vi "Modules - Communications V2-multiple.vi"() -> ()   [LabVIEW 2019]
uses:
  Controls/UDP - Event.ctl
  Controls/UDP - Status.ctl
  Controls/Communications - State.ctl
  Controls/UDP - Command.ctl
  Controls/eFGV States.ctl
  Controls/Communications - Data Structure.ctl
  Controls/FTDI - Communication.ctl
  Controls/Communication - Write Data.ctl
  Controls/UDP - Communication.ctl
  Controls/Global - Hold.vi
  Controls/Global - IP Address.vi
  Controls/Global - Handle.vi
  Controls/Global - Comport.vi
  Controls/Global - Device.vi
  Controls/Global - Data UDP.vi
  Controls/Global - Device Type.vi
  Controls/Global - Unit.vi
  Controls/Global - ADC.vi
  Controls/Global - PID.vi
  Controls/Global - System.vi
  Controls/Global - Test.vi
  Controls/Global - Channel.vi
  Controls/Global - Rendezvous.vi
  Controls/FGV States.ctl
panel:
  out "element":string
  out "UI Loop":errorcluster
  out "UDP CMD.CMD":T1
  out "Feed Error":errorcluster
  out "i Feed Loop":i32
  out "Feed Loop":T2
  out "i CMD Loop":i32
  out "CMD Loop":T2
  out "i UI Loop":i32
  out "UI Loop":T2
  out "CMD Addr":T3
  out "IP":string
  out "IP Registered":string[](array[string])
  out "Array":cluster{"error out":errorcluster, "IP":string}[](array[cluster])
  out "error out":errorcluster
  in  "timeout ms":i32=1000
  out "data out":string
  out "Array 2":T6(array[cluster]) {"Data"."Event" items=["Stop", "Running", "PID", "Up Limit", "Down Limit", "Load Limit"]; "Data"."Status" items=["Stop", "Ramp Up", "Ramp Down", "Jog Up", "Jog Down", "PID Mode", "PID Ramp"]}
  out "UDP Conn ref":refnum<k16>
  out "Stop":bool=TRUE
  out "IP":string[](array[string])
  out "Device":string[](array[string])
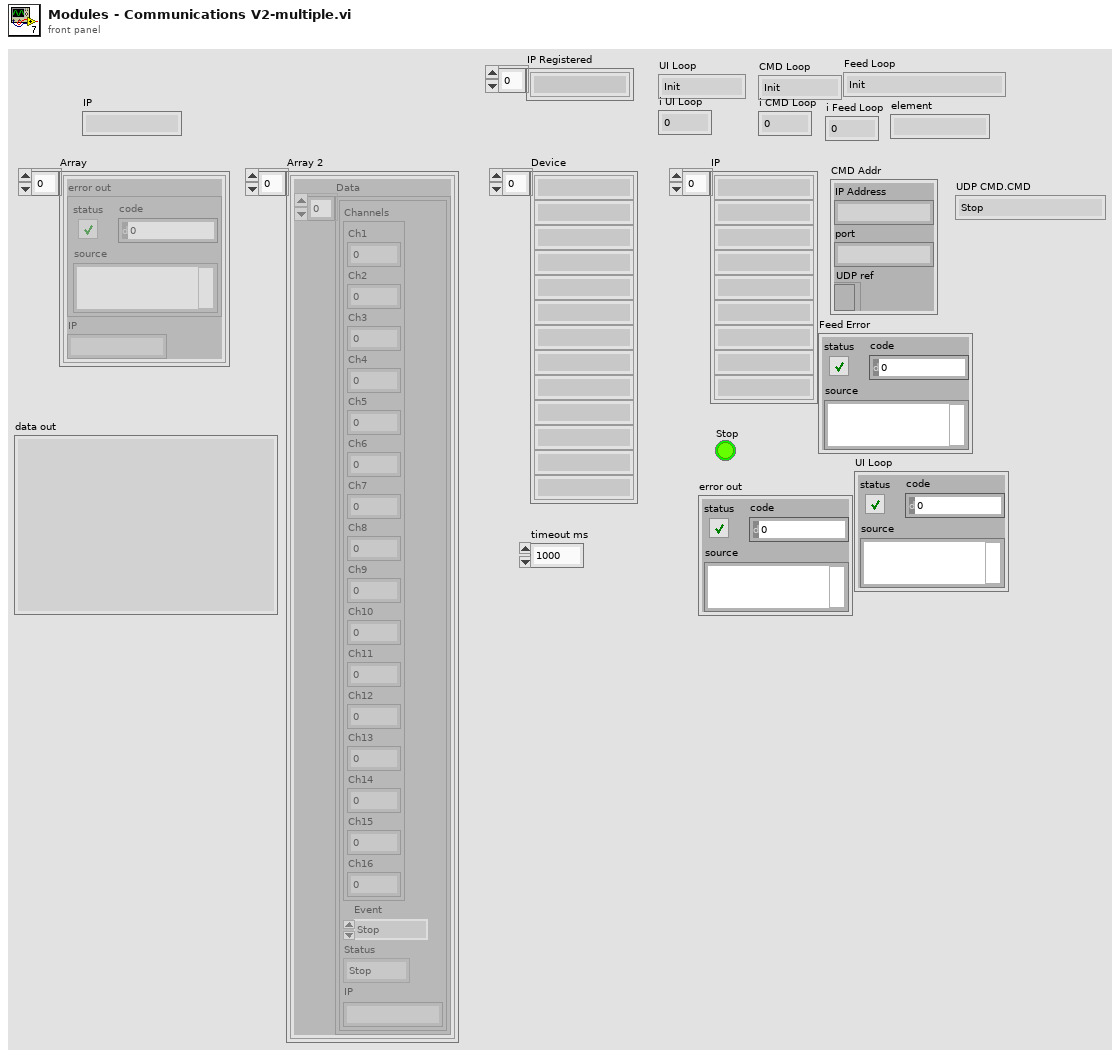
[diagram p1: front panel]
types:
  T1 = typedef "UDP - Command.ctl" = enum16{"Stop", "Jog Up", "Jog Down", "Ramp Up", "Ramp Down", "PID Target", "PID Ramp", "Disp Run", "Read Ch Data", "Zero Channel", "Zero Disp", "Read Sensor", "Write Sensor", "Read ADC", "Write ADC", "Read PID", "Write PID", "Read Test", "Write Test", "Read System", "Write System", "Read Datalog", "Read Datalog Sensor"}
  T2 = typedef "Communications - State.ctl" = enum16{"Init", "Idle", "Command", "Get IP Address", "Release Rendezvous", "Feedback", "Close"}
  T3 = cluster{"IP Address":string, "port":string, "UDP ref":refnum<k16>}
  T4 = typedef "UDP - Event.ctl" = u16
  T5 = typedef "UDP - Status.ctl" = u16
  T6 = cluster{"Data":cluster{"Channels":cluster{"Ch1":sgl, "Ch2":sgl, "Ch3":sgl, "Ch4":sgl, "Ch5":sgl, "Ch6":sgl, "Ch7":sgl, "Ch8":sgl, "Ch9":sgl, "Ch10":sgl, "Ch11":sgl, "Ch12":sgl, "Ch13":sgl, "Ch14":sgl, "Ch15":sgl, "Ch16":sgl}, "Event":T4, "Status":T5, "IP":string}[]}[]
  T7 = cluster{"error out":errorcluster, "name":string}[]
  T8 = enum32{"Invalid", "Standard", "Closed", "Hidden", "Minimized", "Maximized"}
  T9 = typedef "eFGV States.ctl" = enum16{"Init", "Read", "Write", "Exit"}
  T10 = typedef "Communications - Data Structure.ctl" = cluster{"UDP CMD":T11, "Unit?":bool, "Read Unit":bool[], "Trig?":bool, "UDP Info":cluster{"IP Address":string, "port":string, "UDP ref":refnum<k16>}[], "DataLogger":bool[], "VISA Ref":refnum<event-registration>, "Float":sgl, "Data":T12, "UDP Event Ref":refnum<event-registration>, "UDP ref":refnum<k16>, "Read Sensor":u8}
  T11 = typedef "FTDI - Communication.ctl" = cluster{"IP":string, "CMD":T1, "Port":string, "Datalog?":bool, "Float":dbl}
  T12 = typedef "Communication - Write Data.ctl" = cluster{"Test":cluster{"Target Load":sgl, "Target Disp":sgl, "Rate":sgl, "Speed":sgl}, "Sensor":cluster{"Name":string[], "Unit":string[], "Decimal Point":u8[], "Ch Log":u8[], "H Alarm":u8[], "L Alarm":u8[], "H Limit":sgl[], "L Limit":sgl[], "Filter":u8[], "Gain":u8[], "Calib Type":u32[]}, "PID":cluster{"SP":sgl, "PV":sgl, "kP":sgl, "kI":sgl, "kD":sgl, "FF":sgl, "Err Band":sgl, "Max":i32, "Min":i32, "Ts":u32, "Out":i32, "Mode":u8}, "ADC":cluster{"Active Ch":u8[], "Filter Type":u8, "Post Filter":u8[], "Gain":u8[], "FS":u16, "IntOC":u8, "IntFC":u8, "SysOC":u8, "Cofficient":dbl[], "K":dbl[], "Max":i32}, "System":cluster{"Out Type":u8, "Inverse":u8, "Monitor":u8, "Reserve":u8, "ACC Time":u32, "Pulse Rev":u32, "Stroke":u32, "Auto Off":u32, "Gear Ratio":sgl, "Pitch":sgl, "Max Speed":u32, "Jog Speed":u32, "Disp Coff":sgl, "Max Load":u32}, "Index":enum16{"Ch1", "Ch2", "Ch3", "Ch4", "Ch5", "Ch6", "Ch7", "Ch8", "Ch9", "Ch10", "Ch11", "Ch12", "Ch13", "Ch14", "Ch15", "Ch16"}, "Datalog":enum16{"Ch1-Ch16", "Ch17-Ch32", "Ch32-Ch48", "Ch49-Ch64", "Empty"}}
  T13 = enum16{"Ch1-Ch16", "Ch17-Ch32", "Ch32-Ch48", "Ch49-Ch64", "Empty"}
  T14 = cluster{"IP Address":string, "port":string, "UDP ref":refnum<k16>}[]
  T15 = typedef "FGV States.ctl" = enum16{"Read", "Write"}
  T16 = cluster{"Target Load":sgl, "Target Disp":sgl, "Rate":sgl, "Ch4":sgl}
  T17 = cluster{"Name":string[], "Unit":string[], "Decimal Point":u8[], "Ch Log":u8[], "H Alarm":u8[], "L Alarm":u8[], "H Limit":sgl[], "L Limit":sgl[], "Filter":u8[], "Gain":u8[], "Calib Type":u32[]}
  T18 = cluster{"SP":sgl, "PV":sgl, "kP":sgl, "kI":sgl, "kD":sgl, "FF":sgl, "Err Band":sgl, "Max":i32, "Min":i32, "Ts":u32, "Out":i32, "Mode":u8}
  T19 = cluster{"Active Ch":u8[], "Filter Type":u8, "Post Filter":u8[], "Gain":u8[], "FS":u16, "IntOC":u8, "IntFC":u8, "SysOC":u8, "Cofficient":dbl[], "K":dbl[], "Max":i32}
  T20 = cluster{"Out Type":u8, "Inverse":u8, "Monitor":u8, "Reserve":u8, "ACC Time":u32, "Pulse Rev":u32, "Stroke":u32, "Auto Off":u32, "Gear Ratio":sgl, "Pitch":sgl, "Max Speed":u32, "Jog Speed":u32, "Disp Coff":sgl, "Max Load":u32}
  T21 = cluster{"error IO":errorcluster, "name":string}[]
  T22 = cluster{"Name":string[], "Unit":string[], "Decimal Point":u8[], "Ch Log":u8[], "H Alarm":u8[], "L Alarm":u8[], "H Limit":sgl[], "L Limit":sgl[], "Filter":u8[], "Gain":u8[], "Calib Type":u32[]}[]
  T23 = cluster{"Active Ch":u8[], "Filter Type":u8, "Post Filter":u8[], "Gain":u8[], "FS":u16, "IntOC":u8, "IntFC":u8, "SysOC":u8, "Cofficient":dbl[], "K":dbl[], "Max":i32}[]
  T24 = cluster{"SP":sgl, "PV":sgl, "kP":sgl, "kI":sgl, "kD":sgl, "FF":sgl, "Err Band":sgl, "Max":i32, "Min":i32, "Ts":u32, "Out":i32, "Mode":u8}[]
  T25 = cluster{"Out Type":u8, "Inverse":u8, "Monitor":u8, "Reserve":u8, "ACC Time":u32, "Pulse Rev":u32, "Stroke":u32, "Auto Off":u32, "Gear Ratio":sgl, "Pitch":sgl, "Max Speed":u32, "Jog Speed":u32, "Disp Coff":sgl, "Max Load":u32}[]
  T26 = cluster{"Target Load":sgl, "Target Disp":sgl, "Rate":sgl, "Speed":sgl}
  T27 = cluster{"Target Load":sgl, "Target Disp":sgl, "Rate":sgl, "Speed":sgl}[]
  T28 = cluster{"Channels":cluster{"Ch1":sgl, "Ch2":sgl, "Ch3":sgl, "Ch4":sgl, "Ch5":sgl, "Ch6":sgl, "Ch7":sgl, "Ch8":sgl, "Ch9":sgl, "Ch10":sgl, "Ch11":sgl, "Ch12":sgl, "Ch13":sgl, "Ch14":sgl, "Ch15":sgl, "Ch16":sgl}, "Event":T4, "Status":T5, "IP":string}[]
  T29 = cluster{"Data":cluster{"Channels":cluster{"Ch1":sgl, "Ch2":sgl, "Ch3":sgl, "Ch4":sgl, "Ch5":sgl, "Ch6":sgl, "Ch7":sgl, "Ch8":sgl, "Ch9":sgl, "Ch10":sgl, "Ch11":sgl, "Ch12":sgl, "Ch13":sgl, "Ch14":sgl, "Ch15":sgl, "Ch16":sgl}, "Event":T4, "Status":T5, "IP":string}[]}
  T30 = typedef "Rendezvous RefNum" = refnum<k1>
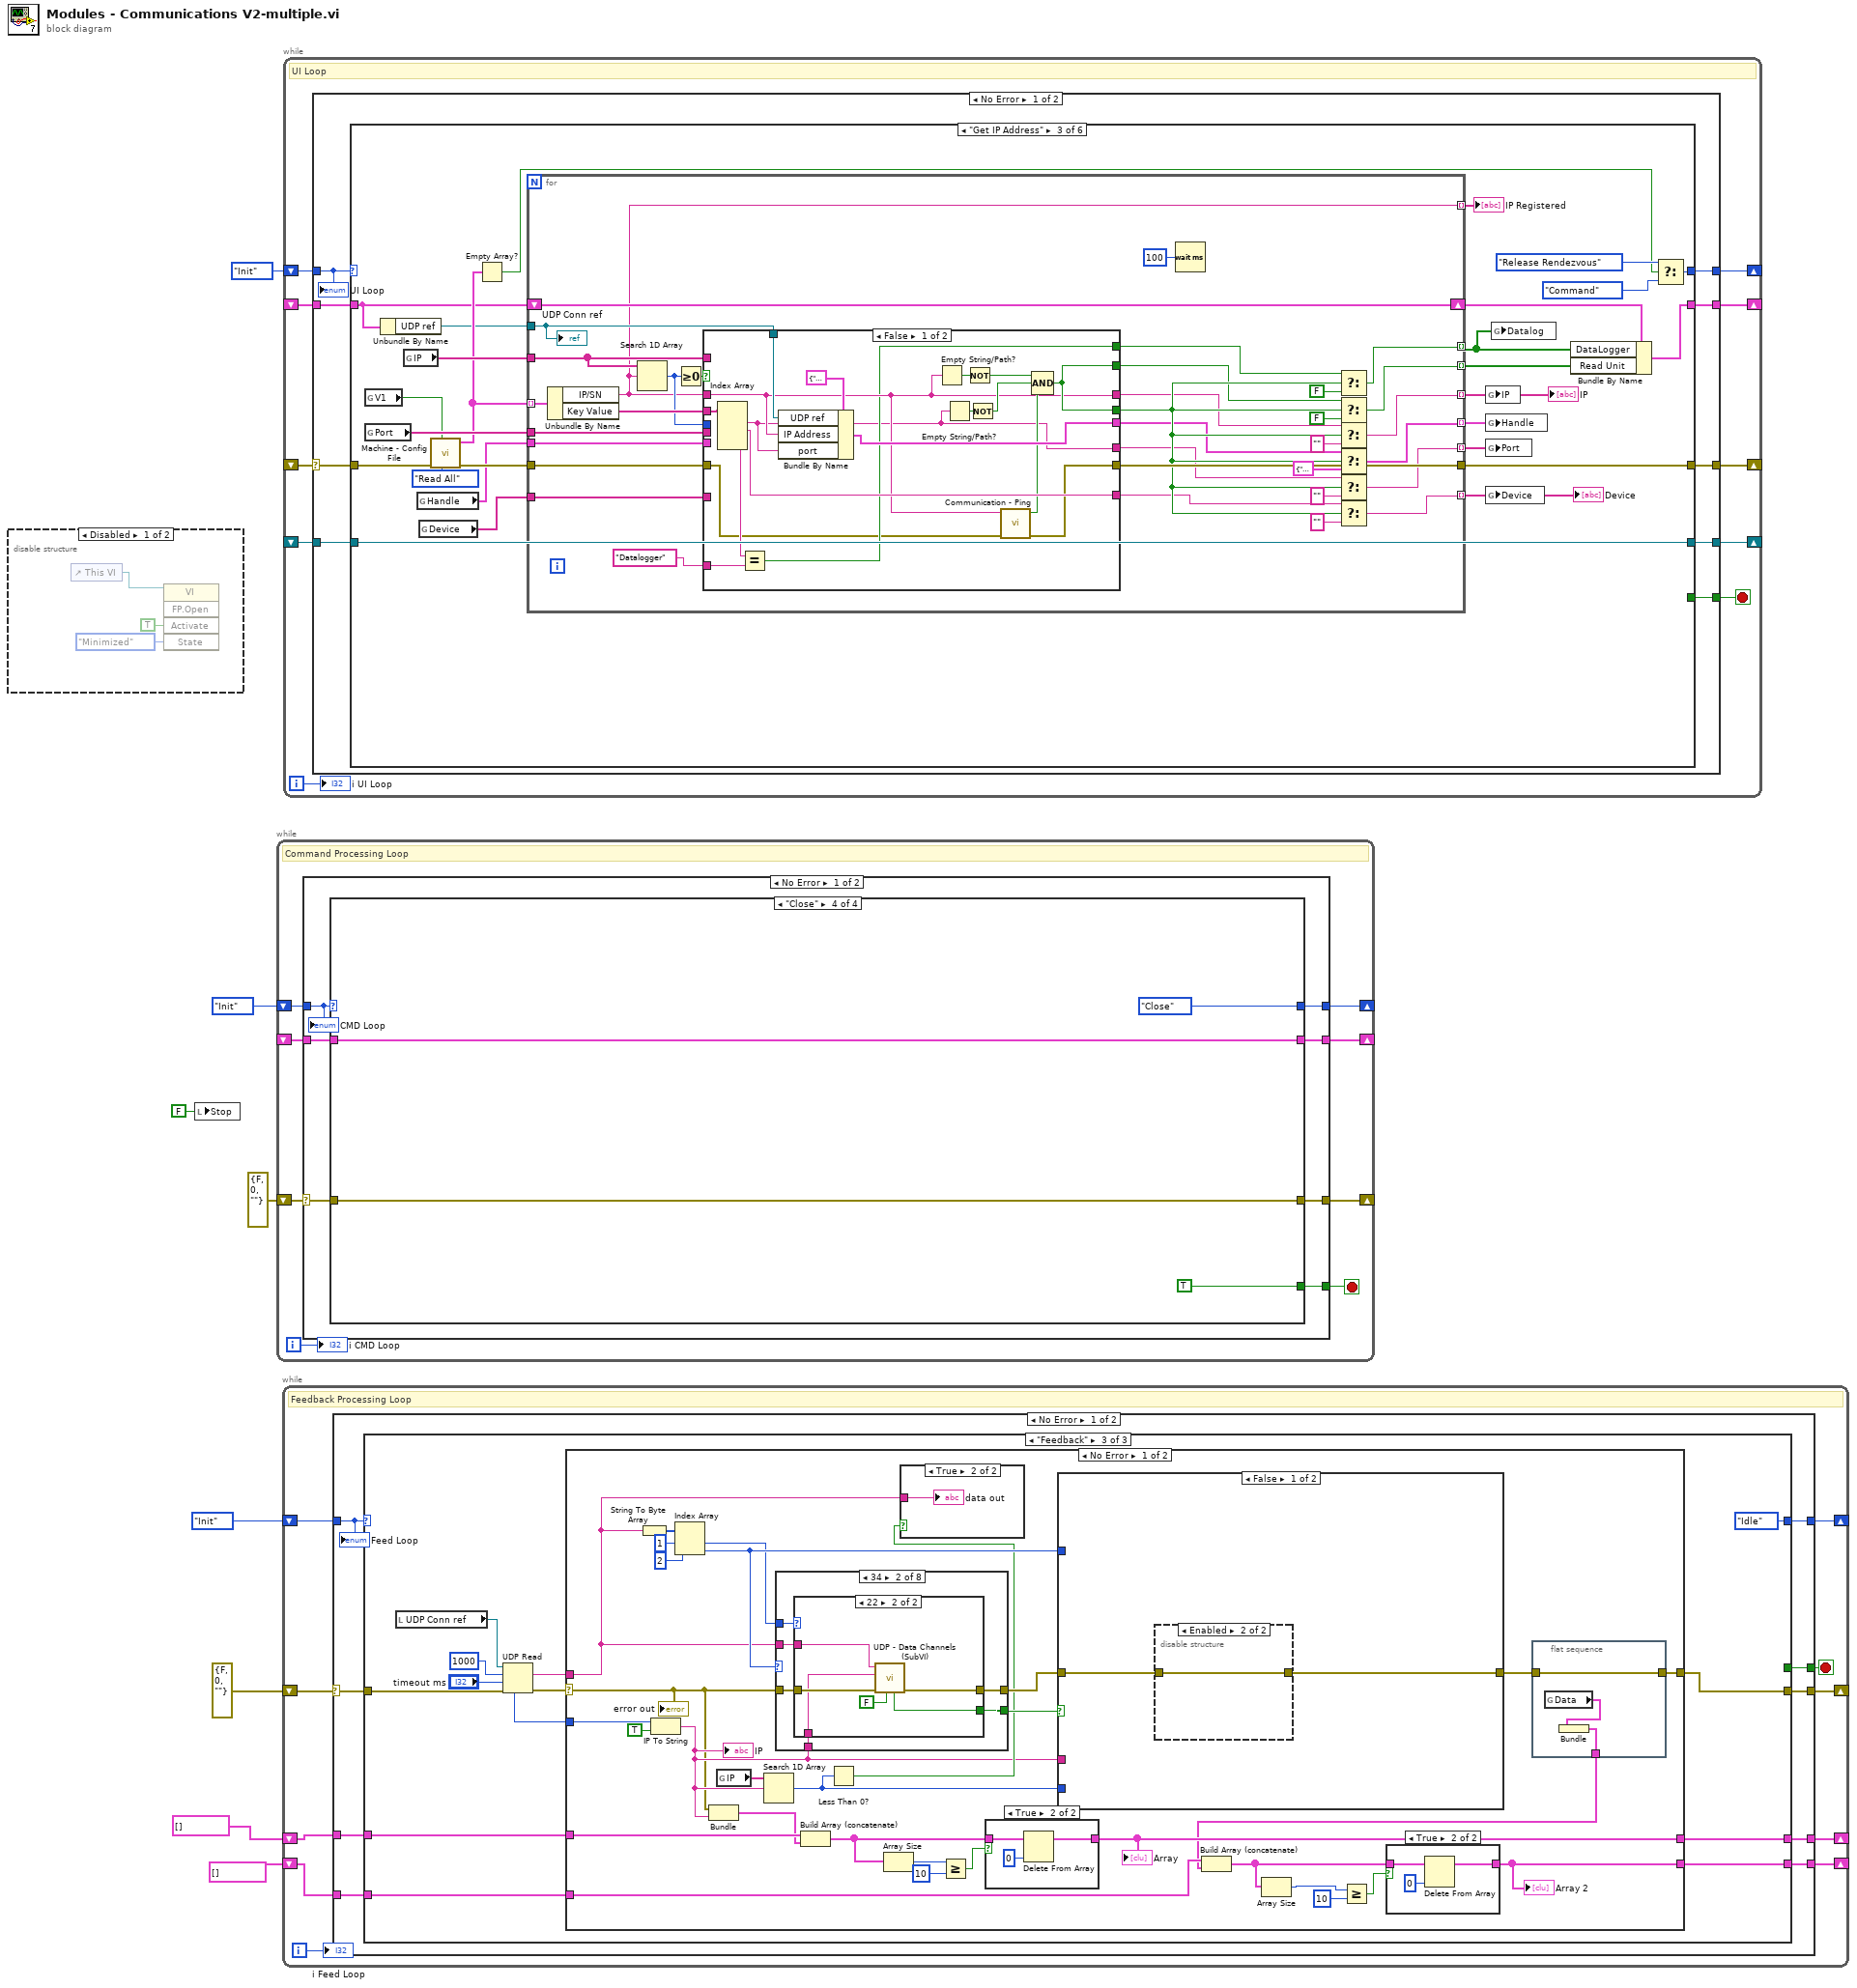
[diagram p0: block diagram]
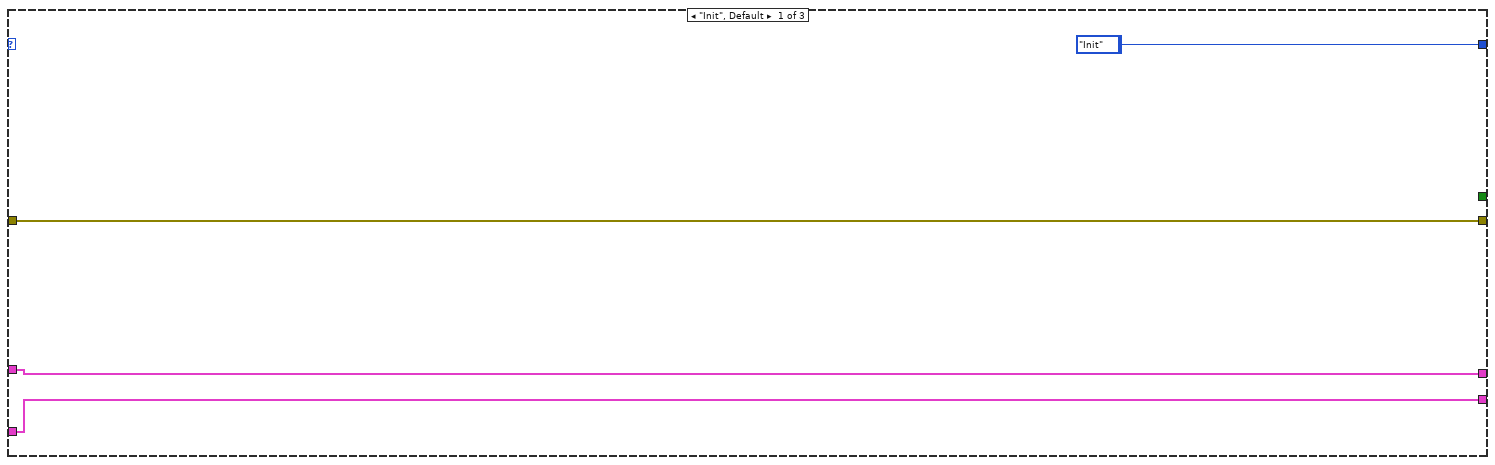
[diagram p3: hidden frame]
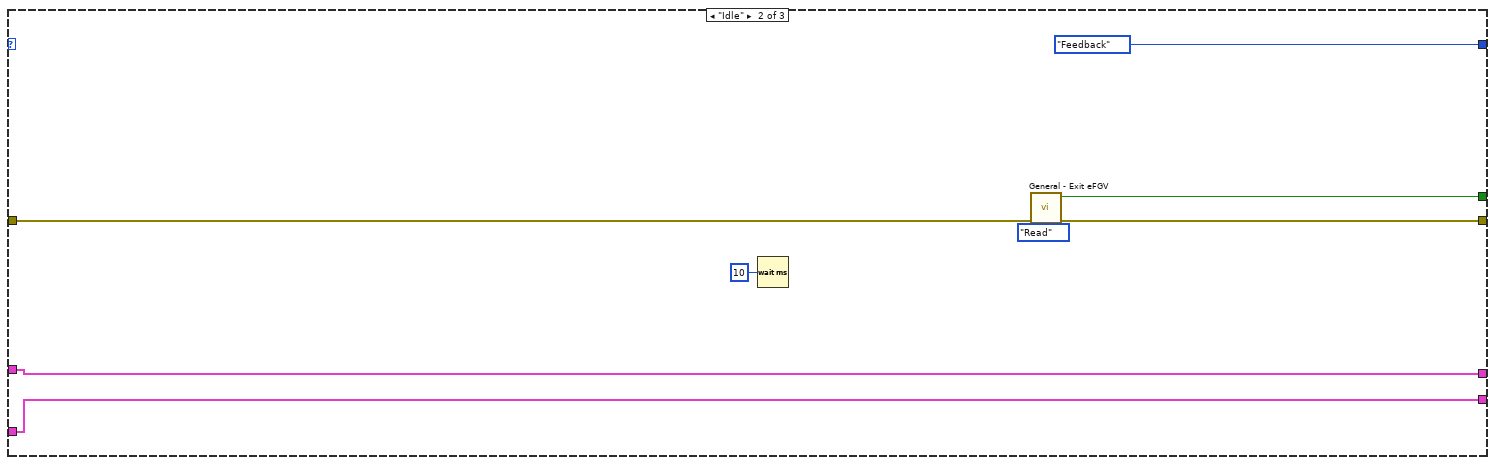
[diagram p4: hidden frame]
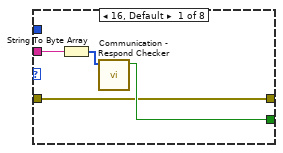
[diagram p8: hidden frame]
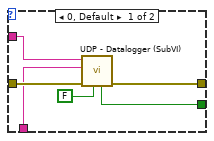
[diagram p9: hidden frame]
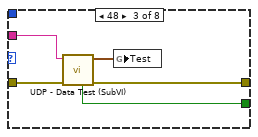
[diagram p10: hidden frame]
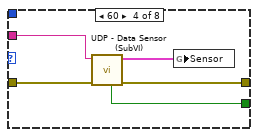
[diagram p11: hidden frame]
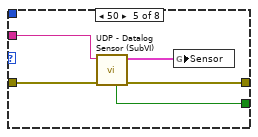
[diagram p12: hidden frame]
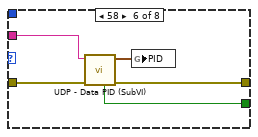
[diagram p13: hidden frame]
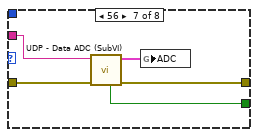
[diagram p14: hidden frame]
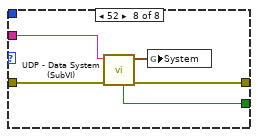
[diagram p15: hidden frame]
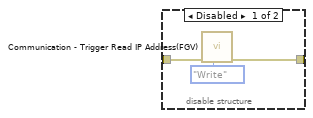
[diagram p16: hidden frame]
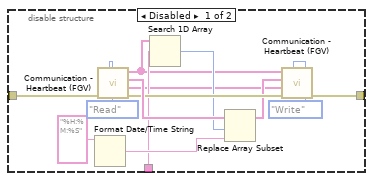
[diagram p19: hidden frame]
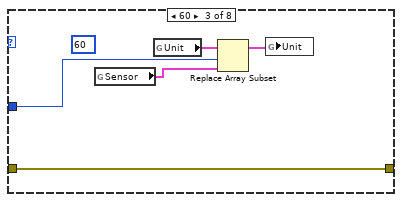
[diagram p20: hidden frame]
diagram:
  (unwired) Communications_-_State."Init"
  (unwired) Communications_-_State."Init"
  n1 = disable-structure shown="Disabled" {
    frame Disabled {
      n2 = control-ref of="This VI"() -> (w11:refnum<vi>)
      n3 = invoke class="VI" method="FP.Open"(reference=w11, "Activate"=TRUE ("Activate?"), "State"=T8."Minimized") -> ()  [unwired: 2 in, 5 out]
    }
    frame Enabled {
    }
  }
  n4 = local write "Stop"(FALSE ("Stop")) -> ()
  n5 = while {
    shift-right: [w18] -> _
    shift-left: errorcluster {"status"=FALSE, "code"=0, "source"=""} ("error IO") -> [w19]
    shift-right: [w16] -> _
    shift-left: Communications_-_State."Init" -> [w17]
    shift-right: [w14] -> _
    shift-left: _ -> [w13]
    i -> [w12]
    stop <- w15 stop-if-true
    # "Command Processing Loop"
    n6 = case shown="No Error" w19 {
      selector: w19 -> [w25 w109]
      tunnel: [w26 w102] -> w18
      tunnel: w17 -> [w24 _]
      tunnel: [w23 Communications_-_State."Idle"] -> w16
      tunnel: [w22 _] -> w15
      tunnel: [w21 w111] -> w14
      tunnel: w13 -> [w20 w111]
      frame No Error {
        n7 = case shown="\"Close\"" w24 {
          tunnel: [w30 w44 w78 w99] -> w26
          tunnel: w25 -> [w28 w43 w88 w99]
          tunnel: [Communications_-_State."Idle" w38 Communications_-_State."Idle" Communications_-_State."Close"] -> w23
          tunnel: [_ _ _ TRUE] -> w22
          tunnel: [w32 w42 w87 w96] -> w21
          tunnel: w20 -> [_ w41 w87 w96]
          frame "Init", Default {
            n8 = call "Communication - UDP Command (eFGV).vi"("Action"=eFGV_States."Read", "error in"=w28) -> ("error out"=w31:errorcluster, "UDP Ref"=w29:refnum<user-event>)  [unwired: 7 in, 1 out]
            n9 = register-events(error in=w31, w29) -> (reference out=w27:refnum<event-registration>, error out=w30:errorcluster)  [unwired: 1 in]
            n10 = Bundle By Name(cluster=T10 {"UDP CMD"={"IP"="", "CMD"=enum."Stop", "Port"="", "Datalog?"=FALSE, "Float"=0.0}, "Unit?"=FALSE, "Read Unit"=[], "Trig?"=FALSE, "UDP Info"=[], "DataLogger"=[], "VISA Ref"=refnum, "Float"=0.0, "Data"={"Test"={"Target Load"=0.0, "Target Disp"=0.0, "Rate"=0.0, "Speed"=0.0}, "Sensor"={"Name"=[], "Unit"=[], "Decimal Point"=[], "Ch Log"=[], "H Alarm"=[], "L Alarm"=[], "H Limit"=[], "L Limit"=[], "Filter"=[], "Gain"=[], "Calib Type"=[]}, "PID"={"SP"=-2.7823365e-08, "PV"=-3.023652e-13, "kP"=8.5432666e-24, "kI"=2.29252e-41, "kD"=1.570387e-38, "FF"=25.0, "Err Band"=0.0, "Max"=15, "Min"=-7, "Ts"=1886611780, "Out"=0, "Mode"=0}, "ADC"={"Active Ch"=[255, 255, 255, 0, 0, 0, 0, 0], "Filter Type"=2, "Post Filter"=[1, 1, 1, 1, 0, 200, 66, 184], "Gain"=[0, 0, 0, 0, 0, 122, 68, 0], "FS"=32, "IntOC"=0, "IntFC"=255, "SysOC"=255, "Cofficient"=[1.0, 1.0, 1.0, 1.0, 1.0, 1.0, 1.0, 1.0], "K"=[1.2450000047683716, 1.2450000047683716], "Max"=1048576}, "System"={"Out Type"=0, "Inverse"=0, "Monitor"=0, "Reserve"=0, "ACC Time"=0, "Pulse Rev"=0, "Stroke"=0, "Auto Off"=0, "Gear Ratio"=0.0, "Pitch"=0.0, "Max Speed"=0, "Jog Speed"=0, "Disp Coff"=0.0, "Max Load"=0}, "Index"=enum."Ch1", "Datalog"=enum."Empty"}, "UDP Event Ref"=refnum, "UDP ref"=refnum, "Read Sensor"=0}, "UDP Event Ref"=w27) -> (w32:T10)
          }
          frame "Idle" {
            n11 = Unbundle By Name(w41) -> ("UDP Event Ref"=w45:refnum<event-registration>)
            n12 = event shown="[0] Timeout" {
              selector: w45 -> [_ _]
              dyn-events: _ -> [_ _]
              timeout: 1000 -> [_ _]
              tunnel: [w51 Communications_-_State."Command" ("f")] -> w39
              tunnel: [w48 w55] -> w44
              tunnel: w43 -> [w48 w55]
              tunnel: [w46 w63] -> w42
              tunnel: w41 -> [w46 w62]
              event Timeout {
                n13 = event-data() -> ()  [unwired: 1 in, 1 out]
                n14 = local read "Stop"() -> (w50:bool)
                n15 = Select(t=Communications_-_State."Close", s=w50, f=Communications_-_State."Idle") -> (s? t:f=w51:T2)
              }
              event User Event {
                n16 = event-data() -> ("IP"=w57:string, "CMD"=w61:T1, "Data"=w52:T12, "Port"=w54:string, "Datalog?"=w53:bool)  [unwired: 1 in]
                n17 = global read "Global - IP Address.vi" "IP"() -> (w60:string[])
                n18 = Index Array(array=w60, index=0) -> (element=w58:string)
                n19 = Equal?(x=w58, y=w57) -> ()  [unwired: 1 out]
                n20 = Bundle By Name(cluster=w62, "UDP CMD.IP"=w57, "UDP CMD.CMD"=w61, "Data"=w52, "UDP CMD.Port"=w54, "UDP CMD.Datalog?"=w53) -> (w63:T10)
              }
            }
            n21 = global read "Global - Hold.vi" "Hold"() -> (w40:bool)
            n22 = Select(t=Communications_-_State."Idle", s=w40, f=w39) -> (s? t:f=w38:T2)
          }
          frame "Command" {
            (unwired) 20
            n23 = Unbundle By Name(w87) -> ("UDP CMD.CMD"=w86:T1, "Data"=w66:T12, "UDP CMD.IP"=w80:string, "UDP CMD.Port"=w74:string, "UDP CMD.Datalog?"=w65:bool)
            "UDP CMD.CMD" <- w86
            n24 = global read "Global - Handle.vi" "Handle"() -> (w82:T14)
            n25 = local read "UDP Conn ref"() -> (w69:refnum<k16>)
            n26 = global read "Global - IP Address.vi" "IP"() -> (w84:string[])
            n27 = Empty String/Path?(string/path=w74) -> (empty?=w75:bool)
            n28 = Search 1D Array(1D array=w84, element=w80) -> (index of element=w68:i32)  [unwired: 1 in]
            n29 = Index Array(array=w82, index=w68) -> (element=w81:T3)
            n30 = Index Array(array=w82, index=w68) -> (element=w79:T3)
            n31 = Unbundle By Name(w81) -> ("UDP ref"=w70:refnum<k16>)
            n32 = Not(x=w75) -> (.not. x?=w71:bool)
            n33 = Unbundle By Name(w79) -> ("port"=w73:string)
            n34 = Select(t=w74, s=w71, f=w73) -> (s? t:f=w72:string)
            n35 = case shown="True" w65 {
              tunnel: w66 -> [w92 w95]
              tunnel: [w91 w94] -> w64
              frame False {
                n36 = Bundle By Name(cluster=w92, "Datalog"=T13."Empty") -> (w91:T12)
              }
              frame True {
                n37 = Bundle By Name(cluster=w95, "Datalog"=T13."Ch1-Ch16") -> (w94:T12)
              }
            }
            n38 = Select(t=w69, s=w71, f=w70) -> (s? t:f=w67:refnum<k16>)
            n39 = Bundle By Name(cluster=T3 {"IP Address"="", "port"="", "UDP ref"=refnum} ("element"), "UDP ref"=w67, "IP Address"=w80, "port"=w72) -> (w77:T3)
            "CMD Addr" <- w77
            n40 = call "UDP - Write CMD.vi"("V2"=TRUE, "CMD"=w86, "error in"=w88, "Data"=w64, "UDP Info"=w77) -> ("error out"=w78:errorcluster)  [unwired: 6 out]
            n41 = Wait (ms)(milliseconds to wait=u32 5) -> ()  [unwired: 1 out]
          }
          frame "Close" {
          }
        }
        "CMD Loop" <- w24
      }
      frame Error {
        n42 = global read "Global - IP Address.vi" "IP"() -> (w108:string[])
        n43 = Unbundle By Name(w109) -> ("source"=w104:string)
        n44 = Index Array(array=w108, index=0) -> (element=w106:string)
        n45 = Concatenate Strings(w106, " - " ("string"), w104) -> (w100:string)
        n46 = call <vilib>:"Clear Errors.vi"("error in (no error)"=w109) -> ("error out"=w103:errorcluster)  [unwired: 5 in, 1 out]
        n47 = call "General - Error Log eFGV.vi"("eFGV States"=eFGV_States."Write", "error in (no error)"=w103, "Error In"=w100) -> ("error out"=w102:errorcluster)  [unwired: 6 in, 2 out]
        n48 = Wait (ms)(milliseconds to wait=u32 100) -> ()  [unwired: 1 out]
      }
    }
    "i CMD Loop" <- w12
  }
  n49 = while {
    shift-right: [w120] -> _
    shift-left: Communications_-_State."Init" -> [w121]
    shift-right: [w119] -> _
    shift-left: errorcluster {"status"=FALSE, "code"=0, "source"=""} ("error IO") -> [w122]
    shift-right: [w117] -> _
    shift-left: T7 [] -> [w116]
    shift-right: [w115] -> _
    shift-left: T6 [] -> [w114]
    i -> [w113]
    stop <- w118 stop-if-true
    # "Feedback Processing Loop"
    n50 = case shown="No Error" w122 {
      selector: w122 -> [w128 w319]
      tunnel: w121 -> [w131 _]
      tunnel: [w130 Communications_-_State."Idle"] -> w120
      tunnel: [w129 w316] -> w119
      tunnel: [w127 _] -> w118
      tunnel: [w126 w315] -> w117
      tunnel: w116 -> [w125 w315]
      tunnel: [w124 w314] -> w115
      tunnel: w114 -> [w123 w314]
      frame No Error {
        n51 = case shown="\"Feedback\"" w131 {
          tunnel: [Communications_-_State."Idle" Communications_-_State."Feedback" Communications_-_State."Idle"] -> w130
          tunnel: [w134 w141 w147] -> w129
          tunnel: w128 -> [w134 w140 w153]
          tunnel: [_ w139 _] -> w127
          tunnel: [w133 w137 w149] -> w126
          tunnel: w125 -> [w133 w137 w150]
          tunnel: [w132 w136 w145] -> w124
          tunnel: w123 -> [w132 w136 w148]
          frame "Init", Default {
            (unwired) Communications_-_State."Init"
          }
          frame "Idle" {
            n52 = Wait (ms)(milliseconds to wait=u32 10) -> ()  [unwired: 1 out]
            n53 = call "General - Exit eFGV.vi"("eFGV States"=eFGV_States."Read", "error in (no error)"=w140) -> ("error out"=w141:errorcluster, "Exit Out"=w139:bool)  [unwired: 7 in, 1 out]
          }
          frame "Feedback" {
            n54 = local read "UDP Conn ref"() -> (w152:refnum<k16>)
            n55 = UDP Read(connection ID=w152, max size (548)=1000, timeout ms (25000)="timeout ms", 8:w153) -> (data out=w151:string, error out=w144:errorcluster, 6:w155:u32)  [unwired: 2 out]
            n56 = case shown="No Error" w144 {
              selector: w144 -> [w157 w313]
              tunnel: w155 -> [w181 _]
              tunnel: w151 -> [w177 _]
              tunnel: w150 -> [w176 w312]
              tunnel: [w172 w312] -> w149
              tunnel: w148 -> [w167 w311]
              tunnel: [w164 w313] -> w147
              tunnel: [w160 w311] -> w145
              frame No Error {
                n57 = String To Byte Array(string=w177) -> (unsigned byte array=w185:u8[])
                n58 = IP To String(1:TRUE ("dot notation? (F)"), 2:w181) -> (0:w159:string)
                "IP" <- w159
                n59 = Index Array(array=w185, index #1=1 ("index"), index #2=2 ("index")) -> (element #1=w186:u8, element #2=w187:u8)
                n60 = Bundle("error IO"=w157, "name"=w159) -> (w158:cluster{"error IO":errorcluster, "name":string})  [unwired: 1 in]
                n61 = global read "Global - IP Address.vi" "IP"() -> (w184:string[])
                n62 = Search 1D Array(1D array=w184, element=w159) -> (index of element=w162:i32)  [unwired: 1 in]
                n63 = case shown="34" w187 {
                  tunnel: [w201 w209 w226 w231 w236 w241 w246 w251] -> w183
                  tunnel: [w202 w208 w225 w230 w235 w240 w245 w250] -> w182
                  tunnel: w157 -> [w201 w205 w223 w228 w233 w238 w243 w248]
                  tunnel: w177 -> [w200 w207 w222 w227 w232 w237 w242 w247]
                  tunnel: w186 -> [_ w206 _ _ _ _ _ _]
                  tunnel: w159 -> [_ w204 _ _ _ _ _ _]
                  frame 16, Default {
                    n64 = String To Byte Array(string=w200) -> (unsigned byte array=w203:u8[])
                    n65 = call "Communication - Respond Checker.vi"("Read Data"=w203) -> ("Success"=w202:bool)  [unwired: 10 in]
                  }
                  frame 34 {
                    n66 = case shown="22" w206 {
                      tunnel: [w213 w221] -> w209
                      tunnel: [w212 w220] -> w208
                      tunnel: w207 -> [w211 w218]
                      tunnel: w205 -> [w214 w217]
                      tunnel: w204 -> [w210 w216]
                      frame 0, Default {
                        n67 = call "UDP - Datalogger (SubVI).vi"("test?"=FALSE, "error in"=w214, "IP"=w210, "data in"=w211) -> ("error out"=w213:errorcluster, "Success"=w212:bool)  [unwired: 5 in, 1 out]
                      }
                      frame 22 {
                        n68 = call "UDP - Data Channels (SubVI).vi"("test?"=FALSE, "error in"=w217, "IP"=w216, "data in"=w218) -> ("error out"=w221:errorcluster, "Success"=w220:bool)  [unwired: 2 in, 4 out]
                      }
                    }
                  }
                  frame 48 {
                    n69 = call "UDP - Data Test (SubVI).vi"("error in"=w223, "data in"=w222) -> ("error out"=w226:errorcluster, "Data Test"=w224:T16, "Success"=w225:bool)  [unwired: 7 in]
                    n70 = global write "Global - Data UDP.vi" "Test"(w224) -> ()
                  }
                  frame 60 {
                    n71 = call "UDP - Data Sensor (SubVI).vi"("error in"=w228, "String"=w227) -> ("error out"=w231:errorcluster, "Sensor Out"=w229:T17, "Success"=w230:bool)  [unwired: 7 in]
                    n72 = global write "Global - Data UDP.vi" "Sensor"(w229) -> ()
                  }
                  frame 50 {
                    n73 = call "UDP - Datalog Sensor (SubVI).vi"("error in"=w233, "String"=w232) -> ("error out"=w236:errorcluster, "Sensor Out"=w234:T17, "Success"=w235:bool)  [unwired: 7 in]
                    n74 = global write "Global - Data UDP.vi" "Sensor"(w234) -> ()
                  }
                  frame 58 {
                    n75 = call "UDP - Data PID (SubVI).vi"("error in (no error)"=w238, "Data"=w237) -> ("error out"=w241:errorcluster, "PID Setting"=w239:T18, "Success"=w240:bool)  [unwired: 7 in]
                    n76 = global write "Global - Data UDP.vi" "PID"(w239) -> ()
                  }
                  frame 56 {
                    n77 = call "UDP - Data ADC (SubVI).vi"("error in (no error)"=w243, "Data"=w242) -> ("error out"=w246:errorcluster, "Data ADC"=w244:T19, "Success"=w245:bool)  [unwired: 7 in]
                    n78 = global write "Global - Data UDP.vi" "ADC"(w244) -> ()
                  }
                  frame 52 {
                    n79 = call "UDP - Data System (SubVI).vi"("error in (no error)"=w248, "Data"=w247) -> ("error out"=w251:errorcluster, "Data System"=w249:T20, "Success"=w250:bool)  [unwired: 7 in]
                    n80 = global write "Global - Data UDP.vi" "System"(w249) -> ()
                  }
                }
                n81 = Build Array (concatenate)(w176, w158) -> (w173:T21)
                n82 = Less Than 0?(x=w162) -> (x < 0?=w161:bool)
                n83 = Array Size(array=w173) -> (size(s)=w175:i32)
                n84 = case shown="True" w161 {
                  tunnel: w177 -> [_ w188]
                  frame False {
                  }
                  frame True {
                    "data out" <- w188
                  }
                }
                n85 = Greater Or Equal?(x=w175, y=10) -> (x >= y?=w171:bool)
                n86 = case shown="True" w171 {
                  tunnel: w173 -> [w196 w199]
                  tunnel: [w196 w198] -> w172
                  frame False {
                  }
                  frame True {
                    n87 = Delete From Array(array=w199, index=0) -> (array with subset deleted=w198:T21)  [unwired: 1 in, 1 out]
                  }
                }
                "Array" <- w172
                n88 = case shown="False" w182 {
                  tunnel: w183 -> [w252 w261]
                  tunnel: [w253 w260] -> w163
                  tunnel: w187 -> [_ w262]
                  tunnel: w162 -> [_ w258]
                  tunnel: w159 -> [_ w259]
                  frame False {
                    n89 = disable-structure shown="Enabled" {
                      disable-tunnel: [w255 w257] -> w253
                      disable-tunnel: w252 -> [w254 w257]
                      frame Disabled {
                        n90 = call "Communication - Trigger Read IP Address(FGV).vi"("Action"=eFGV_States."Write", "error in"=w254) -> ("error out"=w255:errorcluster)  [unwired: 7 in, 2 out]
                      }
                      frame Enabled {
                      }
                    }
                  }
                  frame True {
                    n91 = case shown="34" w262 {
                      tunnel: w261 -> [w263 w266 w282 w287 w292 w300 w305 w310]
                      tunnel: [w263 w265 w282 w287 w292 w300 w305 w310] -> w260
                      tunnel: w258 -> [_ _ w281 w286 w291 w296 w301 w306]
                      tunnel: w259 -> [_ w264 _ _ _ _ _ _]
                      frame 0, Default {
                      }
                      frame 34 {
                        n92 = disable-structure shown="Enabled" {
                          disable-tunnel: w266 -> [w272 w280]
                          disable-tunnel: [w271 w280] -> w265
                          disable-tunnel: w264 -> [w270 _]
                          frame Disabled {
                            n93 = Format Date/Time String(time format string (%c)="%H:%M:%S") -> (date/time string=w276:string)  [unwired: 2 in]
                            n94 = call "Communication - Heartbeat (FGV).vi"("Action"=FGV_States."Read", "error in (no error)"=w272) -> ("error out"=w278:errorcluster, "Previous Out"=w267:string[], "Timestamp Out"=w279:string[], "IP Out"=w268:string[])  [unwired: 6 in]
                            n95 = Search 1D Array(1D array=w268, element=w270) -> (index of element=w269:i32)  [unwired: 1 in]
                            n96 = Replace Array Subset(array=w279, new element=w276, index=w269) -> (w277:string[])
                            n97 = call "Communication - Heartbeat (FGV).vi"("Action"=FGV_States."Write", "error in (no error)"=w278, "Previous"=w267, "Timestamp"=w277, "IP"=w268) -> ("error out"=w271:errorcluster)  [unwired: 3 in, 3 out]
                          }
                          frame Enabled {
                          }
                        }
                      }
                      frame 60 {
                        (unwired) u8 60 ("Numeric")
                        n98 = global read "Global - Data UDP.vi" "Sensor"() -> (w283:T17)
                        n99 = global read "Global - Unit.vi" "Unit"() -> (w284:T22)
                        n100 = Replace Array Subset(array=w284, new element=w283, index=w281) -> (w285:T22)
                        n101 = global write "Global - Unit.vi" "Unit"(w285) -> ()
                      }
                      frame 50 {
                        (unwired) u8 60 ("Numeric")
                        n102 = global read "Global - Data UDP.vi" "Sensor"() -> (w288:T17)
                        n103 = global read "Global - Unit.vi" "Unit"() -> (w289:T22)
                        n104 = Replace Array Subset(array=w289, new element=w288, index=w286) -> (w290:T22)
                        n105 = global write "Global - Unit.vi" "Unit"(w290) -> ()
                      }
                      frame 56 {
                        (unwired) u8 56 ("Numeric")
                        n106 = global read "Global - Data UDP.vi" "ADC"() -> (w293:T19)
                        n107 = global read "Global - ADC.vi" "ADC"() -> (w295:T23)
                        n108 = Replace Array Subset(array=w295, new element=w293, index=w291) -> (w294:T23)
                        n109 = global write "Global - ADC.vi" "ADC"(w294) -> ()
                      }
                      frame 58 {
                        (unwired) u8 58 ("Numeric")
                        n110 = global read "Global - Data UDP.vi" "PID"() -> (w297:T18)
                        n111 = global read "Global - PID.vi" "PID"() -> (w299:T24)
                        n112 = Replace Array Subset(array=w299, new element=w297, index=w296) -> (w298:T24)
                        n113 = global write "Global - PID.vi" "PID"(w298) -> ()
                      }
                      frame 52 {
                        (unwired) u8 52 ("Numeric")
                        n114 = global read "Global - Data UDP.vi" "System"() -> (w302:T20)
                        n115 = global read "Global - System.vi" "System"() -> (w304:T25)
                        n116 = Replace Array Subset(array=w304, new element=w302, index=w301) -> (w303:T25)
                        n117 = global write "Global - System.vi" "System"(w303) -> ()
                      }
                      frame 48 {
                        (unwired) u8 48 ("Numeric")
                        n118 = global read "Global - Data UDP.vi" "Test"() -> (w307:T26)
                        n119 = global read "Global - Test.vi" "Test"() -> (w308:T27)
                        n120 = Replace Array Subset(array=w308, new element=w307, index=w306) -> (w309:T27)
                        n121 = global write "Global - Test.vi" "Test"(w309) -> ()
                      }
                    }
                  }
                }
                n122 = Build Array (concatenate)(w167, w166) -> (w169:T6)
                n123 = Array Size(array=w169) -> (size(s)=w165:i32)
                n124 = Greater Or Equal?(x=w165, y=10) -> (x >= y?=w170:bool)
                n125 = case shown="True" w170 {
                  tunnel: w169 -> [w192 w195]
                  tunnel: [w192 w194] -> w160
                  frame False {
                  }
                  frame True {
                    n126 = Delete From Array(array=w195, index=0) -> (array with subset deleted=w194:T6)  [unwired: 1 in, 1 out]
                  }
                }
                "Array 2" <- w160
                n127 = flat-sequence {
                  tunnel: [w191] -> w166
                  tunnel: [w189] -> w164
                  tunnel: w163 -> [w189]
                  frame #0 {
                    n128 = global read "Global - Channel.vi" "Data"() -> (w190:T28)
                    n129 = Bundle("Data"=w190) -> (w191:T29)  [unwired: 1 in]
                  }
                }
                "error out" <- w157
              }
              frame Error {
                "Feed Error" <- w313
              }
            }
          }
        }
        "Feed Loop" <- w131
      }
      frame Error {
        (unwired) Communications_-_State."Init"
        n130 = call <vilib>:"Clear Errors.vi"("error in (no error)"=w319) -> ("error out"=w316:errorcluster)  [unwired: 5 in, 1 out]
        n131 = Wait (ms)(milliseconds to wait=u32 100) -> ()  [unwired: 1 out]
      }
    }
    "i Feed Loop" <- w113
  }
  n132 = while {
    shift-right: [w328] -> _
    shift-left: _ -> [w329]
    shift-right: [w326] -> _
    shift-left: Communications_-_State."Init" -> [w327]
    shift-right: [w325] -> _
    shift-left: _ -> [w324]
    shift-right: [w322] -> _
    shift-left: _ -> [w321]
    i -> [w320]
    stop <- w323 stop-if-true
    # "UI Loop"
    n133 = case shown="No Error" w329 {
      selector: w329 -> [w337 w576]
      tunnel: [w338 w577] -> w328
      tunnel: w327 -> [w336 w571]
      tunnel: [w335 w571] -> w326
      tunnel: [w334 w582] -> w325
      tunnel: w324 -> [w333 w582]
      tunnel: [w332 _] -> w323
      tunnel: [w331 w581] -> w322
      tunnel: w321 -> [w330 w581]
      frame No Error {
        n134 = case shown="\"Get IP Address\"" w336 {
          tunnel: [w342 w373 w396 w492 w553 w562] -> w338
          tunnel: w337 -> [w354 w372 w407 w495 w552 w561]
          tunnel: [Communications_-_State."Get IP Address" w371 w393 w488 Communications_-_State."Idle" Communications_-_State."Close"] -> w335
          tunnel: [w356 w369 w410 w496 w555 w566] -> w334
          tunnel: w333 -> [_ w370 w410 w496 w555 w566]
          tunnel: [_ _ _ _ _ w564] -> w332
          tunnel: [w349 w368 w397 w486 w550 w563] -> w331
          tunnel: w330 -> [_ w367 w390 w485 w549 w563]
          frame "Init", Default {
            w353 = eFGV_States."Read" ("Action")
            n135 = call "Communication - Trigger Read IP Address(FGV).vi"("Action"=w353, "error in"=w354) -> ("error out"=w355:errorcluster, "Trigger ref"=w352:refnum<user-event>)  [unwired: 7 in, 1 out]
            n136 = call "General - Exit eFGV.vi"("eFGV States"=w353, "error in (no error)"=w355) -> ("error out"=w358:errorcluster, "Exit"=w357:refnum<user-event>)  [unwired: 7 in, 1 out]
            n137 = register-events(error in=w358, w357, w352) -> (reference out=w356:refnum<event-registration>, error out=w350:errorcluster)  [unwired: 1 in]
            n138 = global write "Global - IP Address.vi" "IP"(string[] [] ("IP")) -> ()
            n139 = global write "Global - Comport.vi" "Port"(string[] [] ("Port")) -> ()
            n140 = global write "Global - Device.vi" "Device"(string[] [] ("Device")) -> ()
            n141 = global write "Global - Handle.vi" "Handle"(T14 [] ("Handle")) -> ()
            n142 = Bundle By Name(cluster=T10 {"UDP CMD"={"IP"="", "CMD"=enum."Stop", "Port"="", "Datalog?"=FALSE, "Float"=0.0}, "Unit?"=FALSE, "Read Unit"=[], "Trig?"=FALSE, "UDP Info"=[], "DataLogger"=[], "VISA Ref"=refnum, "Float"=0.0, "Data"={"Test"={"Target Load"=0.0, "Target Disp"=0.0, "Rate"=0.0, "Speed"=0.0}, "Sensor"={"Name"=[], "Unit"=[], "Decimal Point"=[], "Ch Log"=[], "H Alarm"=[], "L Alarm"=[], "H Limit"=[], "L Limit"=[], "Filter"=[], "Gain"=[], "Calib Type"=[]}, "PID"={"SP"=-2.7823365e-08, "PV"=-3.023652e-13, "kP"=8.5432666e-24, "kI"=2.29252e-41, "kD"=1.570387e-38, "FF"=25.0, "Err Band"=0.0, "Max"=15, "Min"=-7, "Ts"=1886611780, "Out"=0, "Mode"=0}, "ADC"={"Active Ch"=[255, 255, 255, 0, 0, 0, 0, 0], "Filter Type"=2, "Post Filter"=[1, 1, 1, 1, 0, 200, 66, 184], "Gain"=[0, 0, 0, 0, 0, 122, 68, 0], "FS"=32, "IntOC"=0, "IntFC"=255, "SysOC"=255, "Cofficient"=[1.0, 1.0, 1.0, 1.0, 1.0, 1.0, 1.0, 1.0], "K"=[1.2450000047683716, 1.2450000047683716], "Max"=1048576}, "System"={"Out Type"=0, "Inverse"=0, "Monitor"=0, "Reserve"=0, "ACC Time"=0, "Pulse Rev"=0, "Stroke"=0, "Auto Off"=0, "Gear Ratio"=0.0, "Pitch"=0.0, "Max Speed"=0, "Jog Speed"=0, "Disp Coff"=0.0, "Max Load"=0}, "Index"=enum."Ch1", "Datalog"=enum."Empty"}, "UDP Event Ref"=refnum, "UDP ref"=refnum, "Read Sensor"=0}, "Read Sensor"=u8 0) -> (w339:T10)
            n143 = global write "Global - Hold.vi" "Hold"(FALSE ("Hold")) -> ()
            n144 = call "UDP - Open Connection.vi"("CMD"=w339, "error in"=w350, "UDP Info"=T3 {"IP Address"="192.168.88.100", "port"="4001", "UDP ref"=refnum}) -> ("error out"=w343:errorcluster, 5:w349:T10)  [unwired: 6 in, 1 out]
            n145 = disable-structure shown="Enabled" {
              disable-tunnel: w343 -> [w363 w365]
              disable-tunnel: [w362 w365] -> w342
              frame Enabled {
                n146 = call <vilib>:"System Exec.vi"("run minimized? (F)"=TRUE, "wait until completion? (T)"=FALSE, "error in (no error)"=w363, "command line"="\"C:\\laragon\\bin\\python\\python-3.10\\python.exe\" \"C:\\laragon\\www\\ping.py\"") -> ("error out"=w362:errorcluster)  [unwired: 4 in, 3 out]
              }
              frame Disabled {
              }
            }
          }
          frame "Idle" {
            n147 = event shown="[1] <Trigger ref>: User Event" {
              selector: w370 -> [_ _ _]
              dyn-events: [_ _ _] -> w369
              timeout: 1000 -> [_ _ _]
              tunnel: [w376 w381 w384] -> w373
              tunnel: w372 -> [w376 w381 w384]
              tunnel: [Communications_-_State."Get IP Address" Communications_-_State."Command" Communications_-_State."Close"] -> w371
              tunnel: [w374 w379 w382] -> w368
              tunnel: w367 -> [w374 w378 w382]
              event Timeout {
                n148 = event-data() -> ()  [unwired: 1 in, 3 out]
              }
              event User Event {
                n149 = event-data() -> ()  [unwired: 1 in, 1 out]
                n150 = Bundle By Name(cluster=w378, "Trig?"=TRUE) -> (w379:T10)
              }
              event User Event {
                n151 = event-data() -> ()  [unwired: 1 in, 5 out]
              }
            }
          }
          frame "Get IP Address" {
            n152 = global read "Global - Data UDP.vi" "V1"() -> (w387:bool)
            n153 = global read "Global - Comport.vi" "Port"() -> (w399:string[])
            n154 = Unbundle By Name(w390) -> ("UDP ref"=w389:refnum<k16>)
            n155 = global read "Global - IP Address.vi" "IP"() -> (w403:string[])
            n156 = global read "Global - Handle.vi" "Handle"() -> (w402:T14)
            n157 = global read "Global - Device.vi" "Device"() -> (w401:string[])
            n158 = call "Machine - Config File.vi"("Action"=enum16{"Write", "Read", "Read All", "Remove"}."Read All", "V1"=w387, "error in (no error)"=w407) -> ("error out"=w408:errorcluster, "Value Out"=w395:cluster{"IP/SN":string, "Key Value":string[]}[])  [unwired: 7 in]
            n159 = Empty Array?(array=w395) -> (empty?=w385:bool)
            n160 = for {
              tunnel: w408 -> [w443]
              tunnel: [w444] -> w396
              tunnel: [w423] -> w406 mode=indexing
              tunnel: [w421] -> w405 mode=indexing
              tunnel: w395 -> [w442] mode=indexing
              tunnel: [w417] -> w404 mode=indexing
              tunnel: w403 -> [w439]
              tunnel: w402 -> [w436]
              tunnel: w401 -> [w438]
              tunnel: [w419] -> w400 mode=indexing
              tunnel: w399 -> [w437]
              tunnel: [w425] -> w398 mode=indexing
              shift-right: [w434] -> w391
              shift-left: w390 -> [w434]
              tunnel: w389 -> [w432]
              tunnel: [w427] -> w388 mode=indexing
              tunnel: [w431] -> w386 mode=indexing
              n161 = Unbundle By Name(w442) -> ("IP/SN"=w431:string, "Key Value"=w441:string[])
              n162 = Search 1D Array(1D array=w439, element=w431) -> (index of element=w435:i32)  [unwired: 1 in]
              n163 = Greater Or Equal To 0?(x=w435) -> (x >= 0?=w440:bool)
              n164 = case shown="False" w440 {
                tunnel: [w452 w475] -> w444
                tunnel: w443 -> [w445 w463]
                tunnel: w441 -> [w461 w473]
                tunnel: [w460 w479] -> w418
                tunnel: [w453 w476] -> w422
                tunnel: [w456 w474] -> w429
                tunnel: w431 -> [w450 _]
                tunnel: [w450 w468] -> w424
                tunnel: w439 -> [_ w482]
                tunnel: w435 -> [_ w478]
                tunnel: w436 -> [_ w481]
                tunnel: w438 -> [_ w480]
                tunnel: [w446 w467] -> w420
                tunnel: w437 -> [_ w477]
                tunnel: [w456 w474] -> w426
                tunnel: w432 -> [w454 _]
                tunnel: "Datalogger" -> [w449 w470]
                tunnel: [w447 w469] -> w428
                frame False {
                  n165 = Index Array(array=w461) -> (element #1=w446:string, element #2=w460:string, element #4=w448:string)  [unwired: 4 in, 1 out]
                  n166 = Equal?(x=w448, y=w449) -> (x = y?=w447:bool)
                  n167 = Bundle By Name(cluster=T3 {"IP Address"="192.168.88.49", "port"="", "UDP ref"=refnum} ("UDP Info"), "UDP ref"=w454, "IP Address"=w450, "port"=w446) -> (w453:T3)
                  n168 = Empty String/Path?(string/path=w450) -> (empty?=w462:bool)
                  n169 = Empty String/Path?(string/path=w446) -> (empty?=w459:bool)
                  n170 = Not(x=w462) -> (.not. x?=w458:bool)
                  n171 = Not(x=w459) -> (.not. x?=w457:bool)
                  n172 = call "Communication - Ping.vi"("error in"=w445, "IP"=w450) -> ("error out"=w452:errorcluster, "Active?"=w451:bool)  [unwired: 7 in, 1 out]
                  n173 = Compound Arithmetic op=AND(w458, w457, w451) -> (w456:bool)
                }
                frame True {
                  n174 = Index Array(array=w480, index=w478) -> (element=w479:string)
                  n175 = Index Array(array=w473, index=3) -> (element=w471:string)
                  n176 = Index Array(array=w482, index=w478) -> (element=w468:string)
                  "element" <- w468
                  n177 = Index Array(array=w481, index=w478) -> (element=w476:T3)
                  n178 = Index Array(array=w477, index=w478) -> (element=w467:string)
                  n179 = Equal?(x=w471, y=w470) -> (x = y?=w469:bool)
                  n180 = call "Communication - Send Command Read.vi"("Datalog?"=w469, "Port"=w467, "Bypass?"=TRUE, "error in (no error)"=w463, "Action"=UDP_-_Command."Read Ch Data", "Device IP Address"=w468) -> ("error out"=w464:errorcluster)  [unwired: 5 in]
                  "UI Loop" <- w464
                  n181 = call "Communication - Ping.vi"("error in"=w464, "IP"=w468) -> ("error out"=w475:errorcluster, "Active?"=w474:bool)  [unwired: 7 in, 1 out]
                }
              }
              n182 = Wait (ms)(milliseconds to wait=u32 100) -> ()  [unwired: 1 out]
              n183 = Select(t=w428, s=w429, f=FALSE) -> (s? t:f=w427:bool)
              n184 = Select(t=w426, s=w429, f=FALSE) -> (s? t:f=w425:bool)
              n185 = Select(t=w424, s=w429, f="") -> (s? t:f=w423:string)
              n186 = Select(t=w422, s=w429, f=T3 {"IP Address"="", "port"="", "UDP ref"=refnum}) -> (s? t:f=w421:T3)
              n187 = Select(t=w420, s=w429, f="") -> (s? t:f=w419:string)
              n188 = Select(t=w418, s=w429, f="") -> (s? t:f=w417:string)
              "UDP Conn ref" <- w432
            }
            "IP" <- w406
            "Device" <- w404
            "IP Registered" <- w386
            n189 = global write "Global - IP Address.vi" "IP"(w406) -> ()
            n190 = global write "Global - Handle.vi" "Handle"(w405) -> ()
            n191 = global write "Global - Comport.vi" "Port"(w400) -> ()
            n192 = global write "Global - Device.vi" "Device"(w404) -> ()
            n193 = global write "Global - Device Type.vi" "Datalog"(w388) -> ()
            n194 = Bundle By Name(cluster=w391, "DataLogger"=w388, "Read Unit"=w398) -> (w397:T10)
            n195 = Select(t=Communications_-_State."Release Rendezvous", s=w385, f=Communications_-_State."Command") -> (s? t:f=w393:T2)
          }
          frame "Command" {
            n196 = Unbundle By Name(w485) -> ("Trig?"=w491:bool, "Read Unit"=w493:bool[], "DataLogger"=w487:bool[], "Read Sensor"=w484:u8)
            n197 = global read "Global - Handle.vi" "Handle"() -> (w494:T14)
            n198 = for {
              shift-right: [w502] -> w492
              shift-left: w495 -> [w503]
              tunnel: w494 -> [w501] mode=indexing
              tunnel: w493 -> [w500] mode=indexing
              tunnel: w487 -> [w499] mode=indexing
              tunnel: w484 -> [w498]
              tunnel: [w497] -> w483
              n199 = case shown="True" w500 {
                tunnel: w503 -> [w505 w511]
                tunnel: [w505 w510] -> w502
                tunnel: w501 -> [_ w509]
                tunnel: w499 -> [_ w508]
                tunnel: w498 -> [w504 w507]
                tunnel: [w504 w506] -> w497
                frame False {
                }
                frame True {
                  n200 = case shown="False" w508 {
                    tunnel: w511 -> [w517 w531]
                    tunnel: [w516 w530] -> w510
                    tunnel: w509 -> [w515 w529]
                    tunnel: w507 -> [w513 w528]
                    tunnel: [w512 w527] -> w506
                    frame False {
                      n201 = case shown="0..5" w513 {
                        selector: w513 -> [w519 w525]
                        tunnel: w517 -> [w524 w526]
                        tunnel: [w523 w526] -> w516
                        tunnel: w515 -> [w521 _]
                        tunnel: [w518 w525] -> w512
                        frame 0..5 {
                          n202 = call "UDP - Write CMD.vi"("V2"=TRUE, "CMD"=UDP_-_Command."Read Sensor", "error in"=w524, "UDP Info"=w521) -> ("error out"=w523:errorcluster)  [unwired: 1 in, 6 out]
                          n203 = Increment(x=w519) -> (x+1=w518:u8)
                        }
                        frame Default {
                        }
                      }
                      n204 = Wait (ms)(milliseconds to wait=u32 10) -> ()  [unwired: 1 out]
                    }
                    frame True {
                      n205 = case shown="0..3" w528 {
                        selector: w528 -> [w533 w547]
                        tunnel: w531 -> [w537 w548]
                        tunnel: [w536 w548] -> w530
                        tunnel: w529 -> [w535 _]
                        tunnel: [w532 w547] -> w527
                        frame 0..3 {
                          n206 = Increment(x=w533) -> (x+1=w532:u8)
                          n207 = for {
                            N: 16 -> [_]
                            tunnel: w535 -> [w543]
                            shift-right: [w545] -> w536
                            shift-left: w537 -> [w546]
                            i -> [w540]
                            n208 = Bundle By Name(cluster=T12 {"Test"={"Target Load"=0.0, "Target Disp"=0.0, "Rate"=0.0, "Speed"=0.0}, "Sensor"={"Name"=[], "Unit"=[], "Decimal Point"=[], "Ch Log"=[], "H Alarm"=[], "L Alarm"=[], "H Limit"=[], "L Limit"=[], "Filter"=[], "Gain"=[], "Calib Type"=[]}, "PID"={"SP"=-2.7823365e-08, "PV"=-3.023652e-13, "kP"=8.5432666e-24, "kI"=2.29252e-41, "kD"=1.570387e-38, "FF"=25.0, "Err Band"=0.0, "Max"=15, "Min"=-7, "Ts"=1886611780, "Out"=0, "Mode"=0}, "ADC"={"Active Ch"=[255, 255, 255, 0, 0, 0, 0, 0], "Filter Type"=2, "Post Filter"=[1, 1, 1, 1, 0, 200, 66, 184], "Gain"=[0, 0, 0, 0, 0, 122, 68, 0], "FS"=32, "IntOC"=0, "IntFC"=255, "SysOC"=255, "Cofficient"=[1.0, 1.0, 1.0, 1.0, 1.0, 1.0, 1.0, 1.0], "K"=[1.2450000047683716, 1.2450000047683716], "Max"=1048576}, "System"={"Out Type"=0, "Inverse"=0, "Monitor"=0, "Reserve"=0, "ACC Time"=0, "Pulse Rev"=0, "Stroke"=0, "Auto Off"=0, "Gear Ratio"=0.0, "Pitch"=0.0, "Max Speed"=0, "Jog Speed"=0, "Disp Coff"=0.0, "Max Load"=0}, "Index"=enum."Ch1", "Datalog"=enum."Empty"} ("Data"), "Index"=w540) -> (w539:T12)
                            n209 = call "UDP - Write CMD.vi"("V2"=TRUE, "CMD"=UDP_-_Command."Read Datalog Sensor", "error in"=w546, "Data"=w539, "UDP Info"=w543) -> ("error out"=w545:errorcluster)  [unwired: 6 out]
                            n210 = Wait (ms)(milliseconds to wait=u32 10) -> ()  [unwired: 1 out]
                          }
                        }
                        frame Default {
                        }
                      }
                    }
                  }
                }
              }
            }
            n211 = Select(t=Communications_-_State."Idle", s=w491, f=Communications_-_State."Release Rendezvous") -> (s? t:f=w488:T2)
            n212 = Bundle By Name(cluster=w485, "Read Sensor"=w483) -> (w486:T10)
          }
          frame "Release Rendezvous" {
            n213 = disable-structure shown="Enabled" {
              disable-tunnel: [w558 w559] -> w553
              disable-tunnel: w552 -> [w557 w559]
              frame Disabled {
                n214 = global read "Global - Rendezvous.vi" "rendezvous"() -> (w556:T30)
                n215 = call <vilib>:"Wait at Rendezvous.vi"("error in (no error)"=w557, "rendezvous"=w556) -> ("error out"=w558:errorcluster)  [unwired: 3 in, 2 out]
              }
              frame Enabled {
              }
            }
            n216 = Bundle By Name(cluster=w549, "Trig?"=TRUE) -> (w550:T10)
          }
          frame "Close" {
            w564 = TRUE
            n217 = global read "Global - Handle.vi" "Handle"() -> (w560:T14)
            n218 = for {
              tunnel: w560 -> [w570] mode=indexing
              shift-right: [w568] -> w562
              shift-left: w561 -> [w569]
              n219 = Unbundle By Name(w570) -> ("UDP ref"=w567:refnum<k16>)
              n220 = UDP Close(connection ID=w567, 8:w569) -> (error out=w568:errorcluster)  [unwired: 1 out]
            }
            "Stop" <- w564
          }
        }
        "UI Loop" <- w336
      }
      frame Error {
        n221 = Unbundle By Name(w576) -> ("source"=w574:string)
        n222 = Concatenate Strings("UI Loop (Comm)" ("string"), " - " ("string"), w574) -> (w572:string)
        n223 = Wait (ms)(milliseconds to wait=u32 100) -> ()  [unwired: 1 out]
        n224 = call <vilib>:"Clear Errors.vi"("error in (no error)"=w576) -> ("error out"=w578:errorcluster)  [unwired: 5 in, 1 out]
        n225 = call "General - Error Log eFGV.vi"("eFGV States"=eFGV_States."Write", "error in (no error)"=w578, "Error In"=w572) -> ("error out"=w577:errorcluster)  [unwired: 6 in, 2 out]
      }
    }
    "i UI Loop" <- w320
  }
